vi "BiggestComplexBlob.vi"(0 "Connectivity":enum16{"4", "8"}(ring)=enum."8", 1 "Image in":T1 {"Dialogs" format="%.0b"}) -> (2 "Centroid":cluster{"X":dbl, "Y":dbl}, 3 "Area":dbl, 4 "Image out":T1 {"Dialogs" format="%.0b"})   [LabVIEW 2024]
doc: "This VI takes a binary image as an input and produces a cluster of X and Y values corresponding to the centroid of the largest contiguous region of pixels (i.e. a “blob”). It also returns a value equal to the area of the region.\n\nTo complete this task, this VI performs a depth-first search on an image to determine the number of blobs. \n\nInput must be a binary image. \n\n<B>Connectivity</B> defines the way in which blobs are searched. 4-connectivity will yield more small blobs, since diagonals are not considered connections. 8-connectivity will yield fewer, larger blobs."
uses:
  <userlib>/ImageProcessing/QTLIB_2595_LV86/QT_Image.ctl
panel:
  # "This VI performs a depth-first search on an image to \ndetermine the number of blobs and returns a parameter\nof  the blob.\n\nInput must be a binary image.  \n\nConnectivity defines the way in which blobs are \nsearched.  4-connectivity will yield more small blobs, \nsince diagonals are not considered connections.\n8-connectivity will yield fewer, larger blobs.  \n\nOutput is an image in which each blob is identified by \na number.  All pixels corresponding to blob #1 are \ngiven the value 1, while all those corresponding to \nblob #2 are given the value 2 and so on.  Also, an array\nof blob sizes indicates the number of blobs\nfound and each of their sizes."
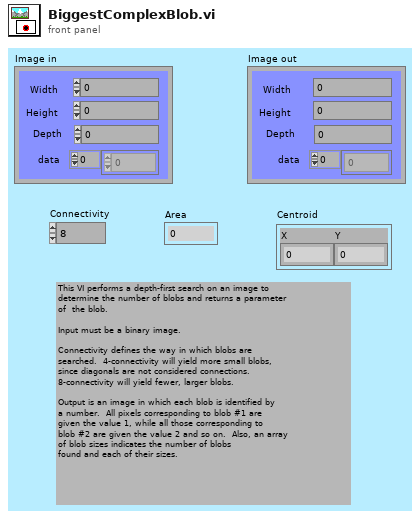
[diagram p1: front panel]
types:
  T1 = typedef "QT_Image.ctl" = cluster{"Width":i32, "Height":i32, "Depth":i32, "data":u8[], "Compressed data":u8[], "Color table":u32[], "Duration":i32, "Options":i32, "Timestamp":i32, "ID":i32, "Reserved":i32, "Dialogs":u32}
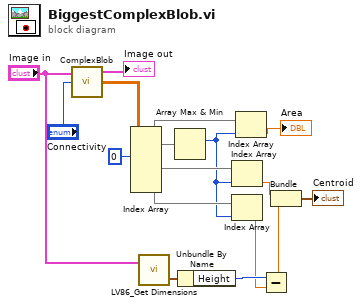
[diagram p0: block diagram]
diagram:
  n1 = call <userlib>:"ComplexBlob.vi"("Connectivity"="Connectivity", "Image in"="Image in") -> ("Parameters"=w14:dbl[][], "Image out"=→"Image out":T1)  [unwired: 1 in, 1 out]
  n2 = Index Array(array=w14, index (col) #1=0 ("disabled index (col)")) -> (element #1=w9:dbl[], element #2=w12:dbl[], element #3=w11:dbl[])  [unwired: 5 in]
  n3 = call <userlib>:"LV86_Get Dimensions.vi"("Image In"="Image in") -> ("Dimensions"=w5:cluster{"Width":i32, "Height":i32})  [unwired: 1 in, 1 out]
  n4 = Array Max & Min(array=w9) -> (max index (indices)=w10:i32)  [unwired: 3 out]
  n5 = Unbundle By Name(w5) -> ("Height"=w3:i32)
  n6 = Index Array(array=w12, index=w10) -> (element=w8:dbl)
  n7 = Index Array(array=w11, index=w10) -> (element=w2:dbl)
  n8 = Index Array(array=w9, index=w10) -> (element=→"Area":dbl)
  n9 = Subtract(x=w3, y=w2) -> (x-y=w1:dbl)
  n10 = Bundle(w8, w1) -> (→"Centroid":cluster{dbl, dbl})  [unwired: 1 in]
